vi "ZCAN_GetDeviceInfo.vi"(0 "DEVICE_HANDLE":u32, 3 "error in (no error)":errorcluster caption="错误输入（无错误）") -> (5 "DEVICE_INFO":string, 6 "SerialNumber":string, 8 "error out":errorcluster caption="错误输出")   [LabVIEW 2020, in "zlgcan.lvlib"]
uses:
  zlgcan.lvlib
  bin/zlgcan_wrap.dll
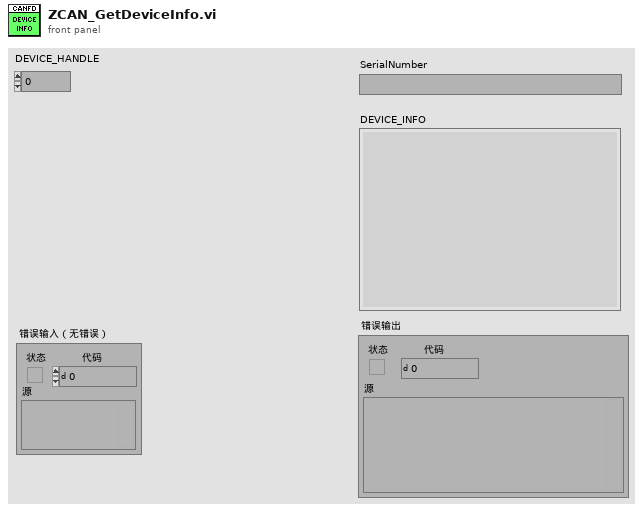
[diagram p1: front panel]
types:
  T1 = cluster{"[0]":u16, "[1]":u16, "[2]":u16, "[3]":u16, "[4]":u16, "[5]":u16, "[6]":u16, "[7]":u16, "[8]":u16, "[9]":u16, "[10]":u16, "[11]":u16, "[12]":u16, "[13]":u16, "[14]":u16, "[15]":u16, "[16]":u16, "[17]":u16, "[18]":u16, "[19]":u16}
  T2 = cluster{"[0]":u16, "[1]":u16, "[2]":u16, "[3]":u16, "[4]":u16, "[5]":u16, "[6]":u16, "[7]":u16, "[8]":u16, "[9]":u16, "[10]":u16, "[11]":u16, "[12]":u16, "[13]":u16, "[14]":u16, "[15]":u16, "[16]":u16, "[17]":u16, "[18]":u16, "[19]":u16, "[20]":u16, "[21]":u16, "[22]":u16, "[23]":u16, "[24]":u16, "[25]":u16, "[26]":u16, "[27]":u16, "[28]":u16, "[29]":u16, "[30]":u16, "[31]":u16, "[32]":u16, "[33]":u16, "[34]":u16, "[35]":u16, "[36]":u16, "[37]":u16, "[38]":u16, "[39]":u16}
  T3 = cluster{"[0]":u16, "[1]":u16, "[2]":u16, "[3]":u16}
  T4 = cluster{u16, u16, u16, u16, u16, u8, cluster{"[0]":u16, "[1]":u16, "[2]":u16, "[3]":u16, "[4]":u16, "[5]":u16, "[6]":u16, "[7]":u16, "[8]":u16, "[9]":u16, "[10]":u16, "[11]":u16, "[12]":u16, "[13]":u16, "[14]":u16, "[15]":u16, "[16]":u16, "[17]":u16, "[18]":u16, "[19]":u16}, cluster{"[0]":u16, "[1]":u16, "[2]":u16, "[3]":u16, "[4]":u16, "[5]":u16, "[6]":u16, "[7]":u16, "[8]":u16, "[9]":u16, "[10]":u16, "[11]":u16, "[12]":u16, "[13]":u16, "[14]":u16, "[15]":u16, "[16]":u16, "[17]":u16, "[18]":u16, "[19]":u16, "[20]":u16, "[21]":u16, "[22]":u16, "[23]":u16, "[24]":u16, "[25]":u16, "[26]":u16, "[27]":u16, "[28]":u16, "[29]":u16, "[30]":u16, "[31]":u16, "[32]":u16, "[33]":u16, "[34]":u16, "[35]":u16, "[36]":u16, "[37]":u16, "[38]":u16, "[39]":u16}, cluster{"[0]":u16, "[1]":u16, "[2]":u16, "[3]":u16}}
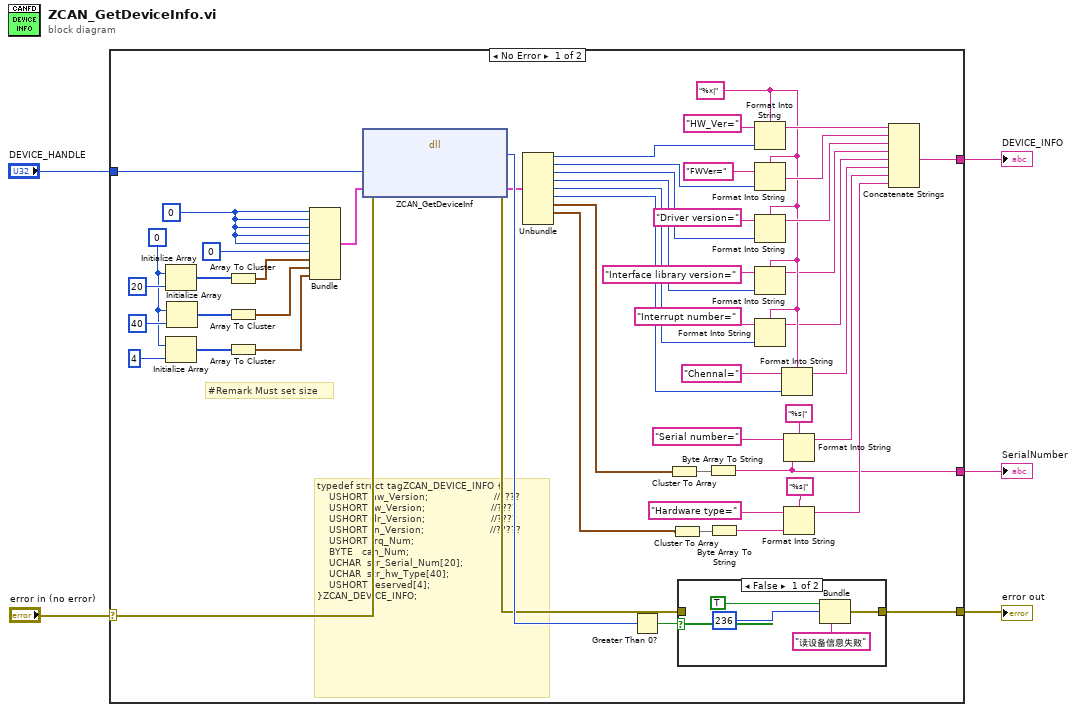
[diagram p0: block diagram]
diagram:
  n1 = case shown="No Error" "error in (no error)" {
    selector: "error in (no error)" -> [w17 w63]
    tunnel: [w54 w63] -> w4
    tunnel: "DEVICE_HANDLE" -> [w57 _]
    tunnel: [w34 _] -> w3
    tunnel: [w18 _] -> w1
    frame No Error {
      w25 = u16 0
      w30 = u16 0
      w40 = "%x|" ("format string")
      # "#Remark Must set size"
      # "typedef struct tagZCAN_DEVICE_INFO {\n    USHORT hw_Version;                      //????\n    USHORT fw_Version;                      //????\n    USHORT dr_Version;                      //????\n    USHORT in_Version;                      //?????\n    USHORT irq_Num;\n    BYTE   can_Num;\n    UCHAR  str_Serial_Num[20];\n    UCHAR  str_hw_Type[40];\n    USHORT reserved[4];\n}ZCAN_DEVICE_INFO;"
      n2 = Initialize Array(w25, 20 ("dimension size")) -> (w15:u16[])
      n3 = Initialize Array(w25, 4 ("dimension size")) -> (w12:u16[])
      n4 = Initialize Array(w25, 40 ("dimension size")) -> (w13:u16[])
      n5 = Array To Cluster(array=w15) -> (cluster=w14:T1)
      n6 = Array To Cluster(array=w13) -> (cluster=w11:T2)
      n7 = Array To Cluster(array=w12) -> (cluster=w10:T3)
      n8 = Bundle(w30, w30, w30, w30, w30, u8 0, w14, w11, w10) -> (w31:T4)  [unwired: 1 in]
      n9 = dll-call lib="E:/Jabil tools/JabilTestLib/ZLG_CANFD/bin/zlgcan_wrap.dll" fn="ZCAN_GetDeviceInf"(error in=w17, "DEVICE_HANDLE"=w57, "pInfo"=w31) -> (error out=w16:errorcluster, "return"=w56:u32, "pInfo"=w53:T4)  [unwired: 3 in, 1 out]
      n10 = Unbundle(w53) -> (w32:u16, w44:u16, w43:u16, w42:u16, w41:u16, w39:u8, w7:T1, w6:T2)  [unwired: 1 out]
      n11 = Greater Than 0?(x=w56) -> (x > 0?=w55:bool)
      n12 = Cluster To Array(cluster=w7) -> (array=w9:u16[])
      n13 = Cluster To Array(cluster=w6) -> (array=w8:u16[])
      n14 = case shown="False" w55 {
        tunnel: [w58 w62] -> w54
        tunnel: w16 -> [_ w62]
        frame False {
          n15 = Bundle("status"=TRUE, "code"=236, "消息"="读设备信息失败") -> (w58:cluster{"status":bool, "code":i32, "消息":string})  [unwired: 1 in]
        }
        frame True {
        }
      }
      n16 = Byte Array To String(unsigned byte array=w9) -> (string=w18:string)
      n17 = Byte Array To String(unsigned byte array=w8) -> (string=w23:string)
      n18 = Format Into String(format string=w40, initial string="HW_Ver=", w32) -> (resulting string=w50:string)  [unwired: 1 in, 1 out]
      n19 = Format Into String(format string=w40, initial string="FWVer=", w44) -> (resulting string=w49:string)  [unwired: 1 in, 1 out]
      n20 = Format Into String(format string=w40, initial string="Driver version=", w43) -> (resulting string=w52:string)  [unwired: 1 in, 1 out]
      n21 = Format Into String(format string=w40, initial string="Interface library version=", w42) -> (resulting string=w38:string)  [unwired: 1 in, 1 out]
      n22 = Format Into String(format string=w40, initial string="Interrupt number=", w41) -> (resulting string=w37:string)  [unwired: 1 in, 1 out]
      n23 = Format Into String(format string=w40, initial string="Chennal=", w39) -> (resulting string=w36:string)  [unwired: 1 in, 1 out]
      n24 = Format Into String(format string="%s|", initial string="Serial number=", w18) -> (resulting string=w19:string)  [unwired: 1 in, 1 out]
      n25 = Format Into String(format string="%s|", initial string="Hardware type=", w23) -> (resulting string=w35:string)  [unwired: 1 in, 1 out]
      n26 = Concatenate Strings(w50, w49, w52, w38, w37, w36, w19, w35) -> (w34:string)
    }
    frame Error {
    }
  }
  "error out" <- w4
  "DEVICE_INFO" <- w3
  "SerialNumber" <- w1
